vi "Init.vi"(8 "error in":errorcluster) -> (0 "error out":errorcluster)   [LabVIEW 2009, in "Main.lvlib"]
doc: "Main initialization VI. Runs on the program startup."
uses:
  Main.lvlib
  CAN/SubVIs/CAN Jaguar Control Mode.ctl
  OWNCAN.lvlib
  FPGA.lvlib
  Servo.lvlib
  Utility.lvlib
  CAN.lvlib
  Drive.lvlib
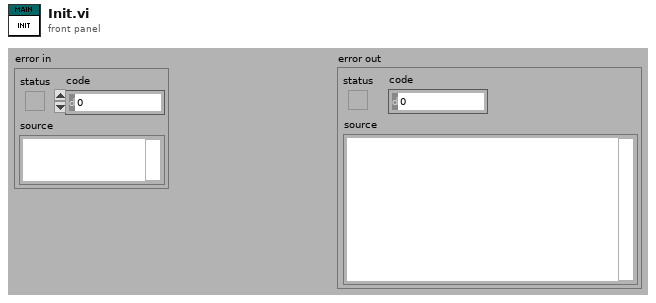
[diagram p1: front panel]
types:
  T1 = typedef "CAN.lvlib/CAN Jaguar Control Mode.ctl" = enum16{"Percent VBus", "Speed", "Position", "Current"}
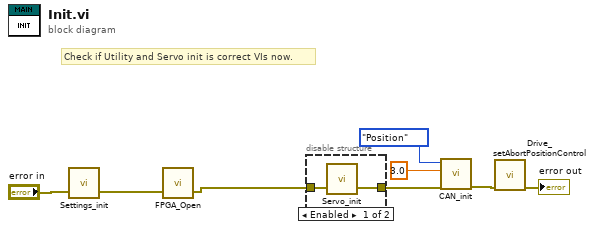
[diagram p0: block diagram]
diagram:
  # "Check if Utility and Servo init is correct VIs now."
  n1 = call "Settings_init.vi"("error in"="error in") -> ("error out"=w8:errorcluster)  [unwired: 2 in]
  n2 = call "FPGA_Open.vi"("error in"=w8) -> ("error out"=w6:errorcluster)  [unwired: 2 in]
  n3 = disable-structure shown="Enabled" {
    disable-tunnel: w6 -> [w10 _]
    disable-tunnel: [w9 _] -> w5
    frame #0 {
      n4 = call "Servo_init.vi"("error in (no error)"=w10) -> ("error out"=w9:errorcluster)  [unwired: 2 in]
    }
    frame #1 {
    }
  }
  n5 = call "CAN_init.vi"("error in"=w5, "Maximum Output Voltage"=3.0, "Control Mode"=CAN_Jaguar_Control_Mode."Position") -> ("error out"=w2:errorcluster)  [unwired: 5 in, 1 out]
  n6 = call "Drive_setAbortPositionControl.vi"("error in (no error)"=w2) -> ("error out"=→"error out":errorcluster)  [unwired: 10 in]
